vi "MC - Fill Default Values.vi"(2 "Key Value In":string[][](array[string]), 3 "Key Name In":string[][](array[string]), 4 "Array of Bad Data":i32[](array[numeric])) -> (0 "Key Value Out":string[][](array[string]), 1 "Key Name Out":string[][](array[string]))   [LabVIEW 2015]
panel:
  in  "Enum":T1(ring)
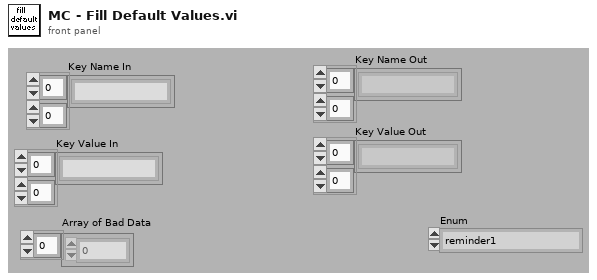
[diagram p1: front panel]
types:
  T1 = enum16{"reminder1", "reminder2", "reminder3", "reminder4", "reminder5", "reminder6", "reminder7", "reminder8", "reminder9", "reminder10"}
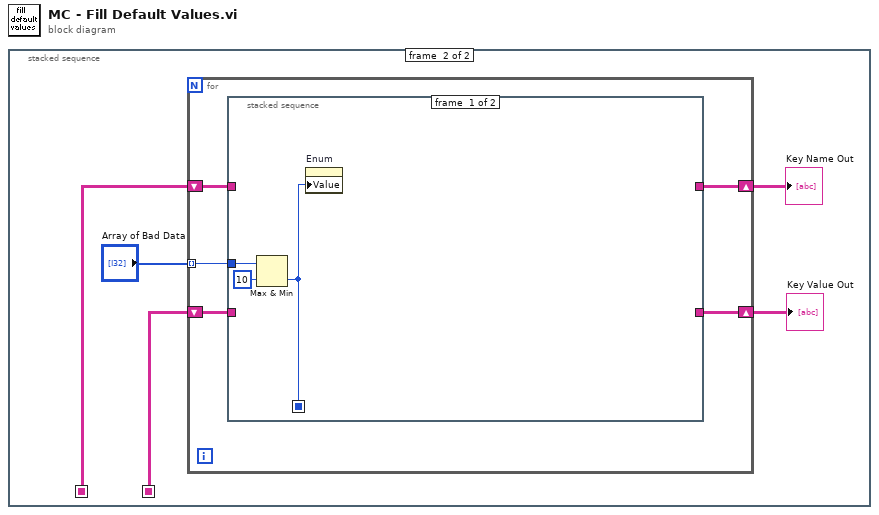
[diagram p0: block diagram]
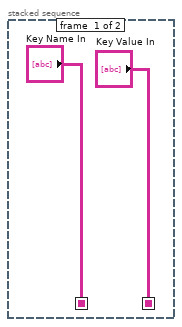
[diagram p2: hidden frame]
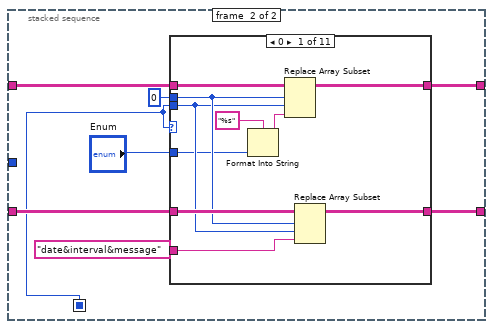
[diagram p3: hidden frame]
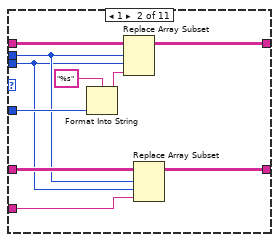
[diagram p4: hidden frame]
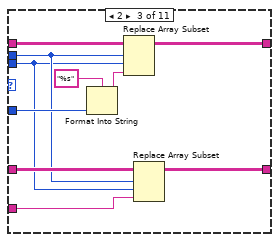
[diagram p5: hidden frame]
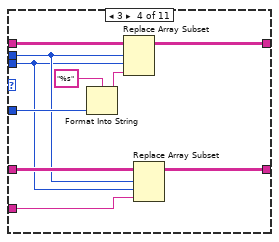
[diagram p6: hidden frame]
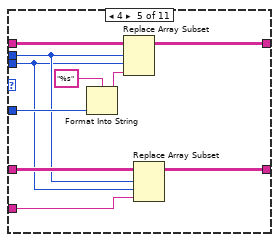
[diagram p7: hidden frame]
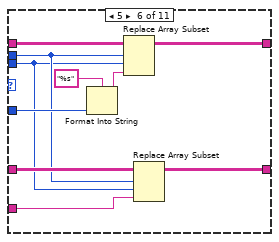
[diagram p8: hidden frame]
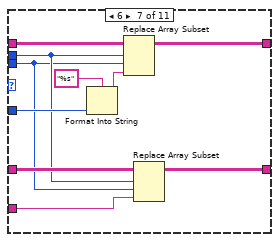
[diagram p9: hidden frame]
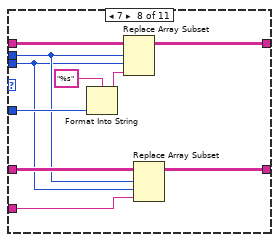
[diagram p10: hidden frame]
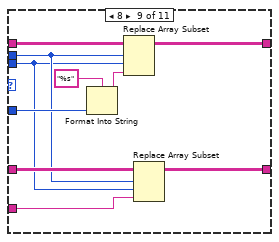
[diagram p11: hidden frame]
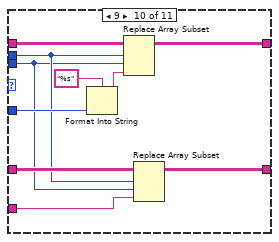
[diagram p12: hidden frame]
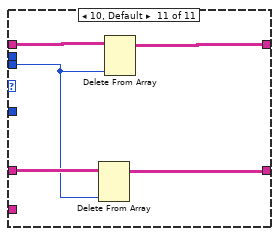
[diagram p13: hidden frame]
diagram:
  n1 = stacked-sequence {
    seq-local: ["Key Name In" _] -> [_ w6]
    seq-local: ["Key Value In" _] -> [_ w5]
    frame #0 {
    }
    frame #1 {
      n2 = for {
        shift-right: [w9] -> w4
        shift-left: w6 -> [w11]
        shift-right: [w12] -> w7
        shift-left: w5 -> [w10]
        tunnel: "Array of Bad Data" -> [w8] mode=indexing
        n3 = stacked-sequence {
          seq-local: [w13 _] -> [_ w16]
          tunnel: [_ w20] -> w12
          tunnel: w11 -> [_ w19]
          tunnel: w10 -> [_ w18]
          tunnel: [_ w17] -> w9
          tunnel: w8 -> [w15 _]
          frame #0 {
            n4 = Max & Min(x=w15, y=10) -> (min(x,y)=w13:i32)  [unwired: 1 out]
            n5 = property on="Enum" class="Enum (strict)"("Value"=w13) -> ()  [unwired: 2 in, 2 out]
          }
          frame #1 {
            n6 = case shown="0" w16 {
              tunnel: w16 -> [w28 w37 w47 w57 w67 w77 w87 w97 w107 w117 w124]
              tunnel: 0 ("Index") -> [w29 w38 w48 w58 w68 w78 w88 w98 w108 w118 _]
              tunnel: w19 -> [w33 w43 w53 w63 w73 w83 w93 w103 w113 w123 w128]
              tunnel: "Enum" -> [w24 w42 w52 w62 w72 w82 w92 w102 w112 w122 _]
              tunnel: w18 -> [w30 w39 w49 w59 w69 w79 w89 w99 w109 w119 w126]
              tunnel: "date&interval&message" -> [w27 w36 w46 w56 w66 w76 w86 w96 w106 w116 _]
              tunnel: [w26 w35 w45 w55 w65 w75 w85 w95 w105 w115 w127] -> w17
              tunnel: [w25 w34 w44 w54 w64 w74 w84 w94 w104 w114 w125] -> w20
              frame 0 {
                n7 = Format Into String(format string="%s", w24) -> (resulting string=w31:string)  [unwired: 2 in, 1 out]
                n8 = Replace Array Subset(array=w33, new element=w31, index (row)=w29, index (col)=w28) -> (w26:string[][])
                n9 = Replace Array Subset(array=w30, new element=w27, index (row)=w29, index (col)=w28) -> (w25:string[][])
              }
              frame 1 {
                n10 = Format Into String(format string="%s", w42) -> (resulting string=w40:string)  [unwired: 2 in, 1 out]
                n11 = Replace Array Subset(array=w43, new element=w40, index (row)=w38, index (col)=w37) -> (w35:string[][])
                n12 = Replace Array Subset(array=w39, new element=w36, index (row)=w38, index (col)=w37) -> (w34:string[][])
              }
              frame 2 {
                n13 = Format Into String(format string="%s", w52) -> (resulting string=w50:string)  [unwired: 2 in, 1 out]
                n14 = Replace Array Subset(array=w53, new element=w50, index (row)=w48, index (col)=w47) -> (w45:string[][])
                n15 = Replace Array Subset(array=w49, new element=w46, index (row)=w48, index (col)=w47) -> (w44:string[][])
              }
              frame 3 {
                n16 = Format Into String(format string="%s", w62) -> (resulting string=w60:string)  [unwired: 2 in, 1 out]
                n17 = Replace Array Subset(array=w63, new element=w60, index (row)=w58, index (col)=w57) -> (w55:string[][])
                n18 = Replace Array Subset(array=w59, new element=w56, index (row)=w58, index (col)=w57) -> (w54:string[][])
              }
              frame 4 {
                n19 = Format Into String(format string="%s", w72) -> (resulting string=w70:string)  [unwired: 2 in, 1 out]
                n20 = Replace Array Subset(array=w73, new element=w70, index (row)=w68, index (col)=w67) -> (w65:string[][])
                n21 = Replace Array Subset(array=w69, new element=w66, index (row)=w68, index (col)=w67) -> (w64:string[][])
              }
              frame 5 {
                n22 = Format Into String(format string="%s", w82) -> (resulting string=w80:string)  [unwired: 2 in, 1 out]
                n23 = Replace Array Subset(array=w83, new element=w80, index (row)=w78, index (col)=w77) -> (w75:string[][])
                n24 = Replace Array Subset(array=w79, new element=w76, index (row)=w78, index (col)=w77) -> (w74:string[][])
              }
              frame 6 {
                n25 = Format Into String(format string="%s", w92) -> (resulting string=w90:string)  [unwired: 2 in, 1 out]
                n26 = Replace Array Subset(array=w93, new element=w90, index (row)=w88, index (col)=w87) -> (w85:string[][])
                n27 = Replace Array Subset(array=w89, new element=w86, index (row)=w88, index (col)=w87) -> (w84:string[][])
              }
              frame 7 {
                n28 = Format Into String(format string="%s", w102) -> (resulting string=w100:string)  [unwired: 2 in, 1 out]
                n29 = Replace Array Subset(array=w103, new element=w100, index (row)=w98, index (col)=w97) -> (w95:string[][])
                n30 = Replace Array Subset(array=w99, new element=w96, index (row)=w98, index (col)=w97) -> (w94:string[][])
              }
              frame 8 {
                n31 = Format Into String(format string="%s", w112) -> (resulting string=w110:string)  [unwired: 2 in, 1 out]
                n32 = Replace Array Subset(array=w113, new element=w110, index (row)=w108, index (col)=w107) -> (w105:string[][])
                n33 = Replace Array Subset(array=w109, new element=w106, index (row)=w108, index (col)=w107) -> (w104:string[][])
              }
              frame 9 {
                n34 = Format Into String(format string="%s", w122) -> (resulting string=w120:string)  [unwired: 2 in, 1 out]
                n35 = Replace Array Subset(array=w123, new element=w120, index (row)=w118, index (col)=w117) -> (w115:string[][])
                n36 = Replace Array Subset(array=w119, new element=w116, index (row)=w118, index (col)=w117) -> (w114:string[][])
              }
              frame 10, Default {
                n37 = Delete From Array(array=w126, index (col)=w124) -> (array with subset deleted=w125:string[][])  [unwired: 2 in, 1 out]
                n38 = Delete From Array(array=w128, index (col)=w124) -> (array with subset deleted=w127:string[][])  [unwired: 2 in, 1 out]
              }
            }
          }
        }
      }
      "Key Name Out" <- w4
      "Key Value Out" <- w7
    }
  }
